vi "tio32_RunMnemo.vi"(0 "VISA resource name":refnum<visa-resource-name>, 1 "Device address":i32=4660 format="%x", 3 "command string":string, 5 "error in (no error)":errorcluster) -> (6 "result count":i32, 8 "result-array":u8[](array[numeric]) format="%x", 10 "ACKS count":i32, 11 "data count":i32, 12 "ACKS-array":u8[](array[numeric]) format="%x", 13 "pData array":i8[](array[numeric])=[48, 32, 48, 32, 48, 32, 48, 0, 0, 0, 0, 0, 0, 0, 0, 0, 0, 0, 0, 0, 0, 0, 0, 0, 0, 0, 0, 0, 0, 0, 0, 0, 0, 0, 0, 0, 0, 0, 0, 0, 0, 0, 0, 0, 0, 0, 0, 0, 0, 0, 0, 0, 0, 0, 0, 0, 0, 0, 0, 0, 0, 0, 0, 0, 0, 0, 0, 0, 0, 0, 0, 0, 0, 0, 0, 0, 0, 0, 0, 0, 0, 0, 0, 0, 0, 0, 0, 0, 0, 0, 0, 0, 0, 0, 0, 0, 0, 0, 0, 0, 0, 0, 0, 0, 0, 0, 0, 0, 0, 0, 0, 0, 0, 0, 0, 0, 0, 0, 0, 0, 0, 0, 0, 0, 0, 0, 0, 0, 0, 0, 0, 0, 0, 0, 0, 0, 0, 0, 0, 0, 0, 0, 0, 0, 0, 0, 0, 0, 0, 0, 0, 0, 0, 0, 0, 0, 0, 0, 0, 0, 0, 0, 0, 0, 0, 0, 0, 0, 0, 0, 0, 0, 0, 0, 0, 0, 0, 0, 0, 0, 0, 0, 0, 0, 0, 0, 0, 0, 0, 0, 0, 0, 0, 0, 0, 0, 0, 0, 0, 0, 0, 0, 0, 0, 0, 0, 0, 0, 0, 0, 0, 0, 0, 0, 0, 0, 0, 0, 0, 0, 0, 0, 0, 0, 0, 0, 0, 0, 0, 0, 0, 0, 0, 0, 0, 0, 0, 0, 0, 0, 0, 0, 0, 0, 0, 0, 0, 0, 0, 0, 0, 0, 0, 0, 0, 0] format="%x", 14 "VISA resource name out":refnum<visa-resource-name>, 15 "return":i32=666, 17 "Tx-Array":u8[](array[numeric]) format="%x", 18 "pRx array":i8[](array[numeric])=[0, -104, 0, 16, 0, 51, 0, 33, 0, 0, 0, 0, 0, 0, 0, 0, 0, 0, 0, 0, 0, 0, 0, 0, 0, 0, 0, 0, 0, 0, 0, 0] format="%x", 19 "error out":errorcluster)   [LabVIEW 2011]
uses:
  l_pse_dll/Tio32.dll
panel:
  out "ACKS display":string
  out "Result display":string
  out "data string display":string
  out "receive string display":string
  out "transmit string display":string
  # "tio32_RunMnemo"
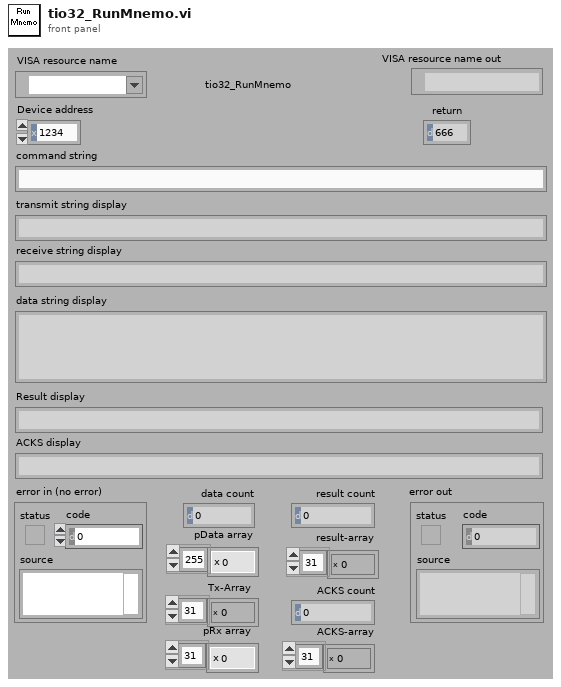
[diagram p1: front panel]
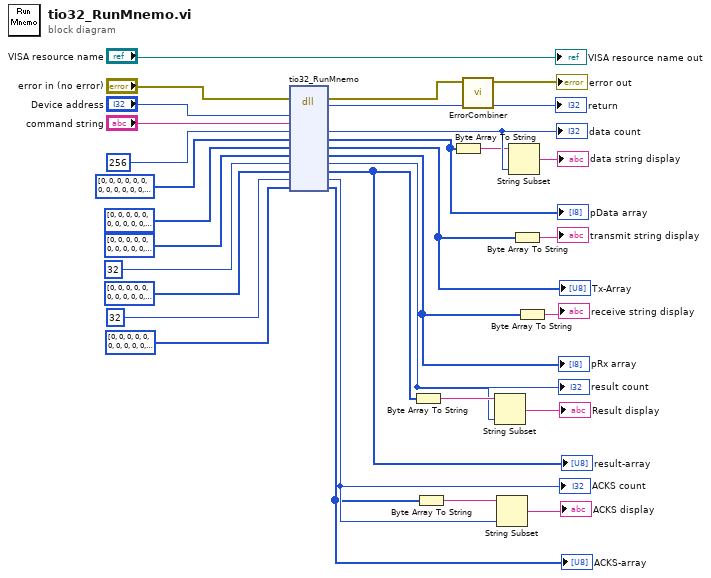
[diagram p0: block diagram]
diagram:
  n1 = dll-call lib="C:/Users/Ikaika's/Documents/DCC/Apps/INA231/INA231-SFT-rev1/INA231-Sourcecode-rev1/INA231/Shell Resources/l_pse_dll/Tio32.dll" fn="tio32_RunMnemo"(error in="error in (no error)", "adr"="Device address", "pCmd"="command string", "dlen"=256, "pdata"=u8[] [0, 0, 0, 0, 0, 0, 0, 0, 0, 0, 0, 0, 0, 0, 0, 0, 0, 0, 0, 0, 0, 0, 0, 0, 0, 0, 0, 0, 0, 0, 0, 1, 0, 0, 0, 0, 0, 0, 0, 0, 0, 0, 0, 0, 0, 0, 0, 0, 0, 0, 0, 0, 0, 0, 0, 0, 0, 0, 0, 0, 0, 0, 0, 0, 0, 0, 0, 0, 0, 0, 0, 0, 0, 0, 0, 0, 0, 0, 0, 0, 0, 0, 0, 0, 0, 0, 0, 0, 0, 0, 0, 0, 0, 0, 0, 0, 0, 0, 0, 0, 0, 0, 0, 0, 0, 0, 0, 0, 0, 0, 0, 0, 0, 0, 0, 0, 0, 0, 0, 0, 0, 0, 0, 0, 0, 0, 0, 0, 0, 0, 0, 0, 0, 0, 0, 0, 0, 0, 0, 0, 0, 0, 0, 0, 0, 0, 0, 0, 0, 0, 0, 0, 0, 0, 0, 0, 0, 0, 0, 0, 0, 0, 0, 0, 0, 0, 0, 0, 0, 0, 0, 0, 0, 0, 0, 0, 0, 0, 0, 0, 0, 0, 0, 0, 0, 0, 0, 0, 0, 0, 0, 0, 0, 0, 0, 0, 0, 0, 0, 0, 0, 0, 0, 0, 0, 0, 0, 0, 0, 0, 0, 0, 0, 0, 0, 0, 0, 0, 0, 0, 0, 0, 0, 0, 0, 0, 0, 0, 0, 0, 0, 0, 0, 0, 0, 0, 0, 0, 0, 0, 0, 0, 0, 0, 0, 0, 0, 0, 0, 0, 0, 0, 0, 0, 0, 0] ("pTx"), "pTx"=u8[] [0, 0, 0, 0, 0, 0, 0, 0, 0, 0, 0, 0, 0, 0, 0, 0, 0, 0, 0, 0, 0, 0, 0, 0, 0, 0, 0, 0, 0, 0, 0, 0], "pRx"=u8[] [0, 0, 0, 0, 0, 0, 0, 0, 0, 0, 0, 0, 0, 0, 0, 0, 0, 0, 0, 0, 0, 0, 0, 0, 0, 0, 0, 0, 0, 0, 0, 0], "reslen"=i16 32 ("resLen"), "pres"=u8[] [0, 0, 0, 0, 0, 0, 0, 0, 0, 0, 0, 0, 0, 0, 0, 0, 0, 0, 0, 0, 0, 0, 0, 0, 0, 0, 0, 0, 0, 0, 0, 0] ("pRes"), "acklen"=i16 32 ("ackLen"), "pack"=u8[] [0, 0, 0, 0, 0, 0, 0, 0, 0, 0, 0, 0, 0, 0, 0, 0, 0, 0, 0, 0, 0, 0, 0, 0, 0, 0, 0, 0, 0, 0, 0, 0] ("pAck")) -> (error out=w19:errorcluster, "Rückgabetyp"=w18:i32, "dlen"=w23:i32, "pdata"=w24:u8[], "pTx"=w9:u8[], "pRx"=w29:u8[], "reslen"=w12:i32, "pres"=w8:u8[], "acklen"=w11:i32, "pack"=w6:u8[])  [unwired: 4 in, 1 out]
  "pRx array" <- w29
  "data count" <- w23
  "pData array" <- w24
  "result count" <- w12
  "ACKS count" <- w11
  "Tx-Array" <- w9
  "result-array" <- w8
  "ACKS-array" <- w6
  n2 = Byte Array To String(unsigned byte array=w8) -> (string=w13:string)
  n3 = Byte Array To String(unsigned byte array=w6) -> (string=w10:string)
  n4 = Byte Array To String(unsigned byte array=w24) -> (string=w22:string)
  n5 = call "ErrorCombiner.vi"("Return In"=w18, "error in (no error)"=w19) -> ("Return Out"=→"return":i32, "error out"=→"error out":errorcluster)  [unwired: 8 in]
  n6 = String Subset(string=w13, length (rest)=w12) -> (substring=→"Result display":string)  [unwired: 1 in]
  n7 = String Subset(string=w10, length (rest)=w11) -> (substring=→"ACKS display":string)  [unwired: 1 in]
  n8 = String Subset(string=w22, length (rest)=w23) -> (substring=→"data string display":string)  [unwired: 1 in]
  n9 = Byte Array To String(unsigned byte array=w9) -> (string=→"transmit string display":string)
  n10 = Byte Array To String(unsigned byte array=w29) -> (string=→"receive string display":string)
  "VISA resource name out" <- "VISA resource name"
